vi "config Talon FX.vi"(5 "Reverse Limit switch":T12=enum."Normally Closed", 6 "LIMIT SW\nEnabled?":bool, 7 "Forward Limit switch":T12=enum."Normally Closed", 8 "error in (no error)":errorcluster, 11 "Talon FX motor defaults":T6={"refnum name"="ref DRIVE", "CAN ID"=0, "Installed?"=FALSE, "description"="", "MOTOR SELECT"=0, "CAN Bus"="", "Invert Type"=enum."Counter-Clockwise", "Neutral Mode"=enum."EEPROMSetting", "gear ratio"=0.0, "MOTOR PIDF coefficients"={"PIDF"={"P Gain"=0.001, "I Gain"=0.0, "D Gain"=0.0, "F Gain"=0.0012, "I Zone"=0.0, "Min Output"=-1.0, "Max Output"=1.0}, "Smart Motion"={"Max Velocity"=1900.0, "Max Acceleration"=750.0, "Minimum Velocity Output"=0.1, "Allowed Closed Loop Error"=0.02}}, "Throttle"={"Ramp Open (s)"=0.0, "Ramp Closed (s)"=0.0, "Percent Deadband"=0.0}, "Supply Current Limits"={"Enable?"=FALSE, "Current Limit"=0.0, "Threshold Current"=0.0, "Threshold Time"=0.0}} {"gear ratio" format="%_5f"; "MOTOR SELECT" items=["REV NEO"=5676, "REV NEO 550"=11000, "VEX Falcon"=6380, "WC Kraken"=6000]}) -> (0 "error out":errorcluster, 3 "PhoenixMotorControlDevRef":T1={"DeviceStatus"={"status"=FALSE, "code"=0, "source"=""}, "Type"=enum."PWM", "PWM"={"PWM Channel"=enum."Invalid", "DeadBand"={"Name"="", "maxPositivePwm"=0, "minPositivePwm"=0, "centerPwm"=0, "maxNegativePwm"=0, "minNegativePwm"=0, "angularRange"=0}}, "CAN"={"Device Number"=0, "SetOutput VI Ref"=variant(enum8{"Percent VBus", "Current", "Speed", "Position", "Voltage"} enum."Percent VBus"), "GetOutput VI Ref"=variant(refnum<k1> refnum), "Enable VI Ref"=variant(dbl 12.0), "Disable VI Ref"=variant(enum8{"Percent VBus", "Speed", "Position", "Slave", "Unchanged / Invalid", "Voltage Compensation", "Current", "Motion Profile"} enum."Percent VBus"), "Data"=variant}, "Invert"=FALSE, "DIO PWM"={"PWM \"Enable\" Channel"=enum."Invalid", "DIOChannel"=enum."Invalid", "PWM Rate"=0.0}})   [LabVIEW 2023]
uses:
  ctrl defs/ctrl MOTOR SELECT.ctl
  ctrl defs/ctrl motor PIDF coefficients.ctl
  <vilib>/Rock Robotics/WPI/ThirdParty/REV Robotics/REVLib/Typedef/Spark MAX Smart Motion Parameters.ctl
  <vilib>/Rock Robotics/WPI/ThirdParty/REV Robotics/REVLib/Typedef/Spark MAX Limit Switch Polarity.ctl
  <vilib>/Rock Robotics/WPI/ThirdParty/Phoenix-LabVIEW/Motor Controller/Controls/CTRE_Phoenix_MotorControl_FeedbackDevice_TalonFX.ctl
  <vilib>/Rock Robotics/WPI/ThirdParty/Phoenix-LabVIEW/Motor Controller/Controls/CTRE_Phoenix_MotorControl_TalonFXInvertType.ctl
  <vilib>/Rock Robotics/WPI/ThirdParty/Phoenix-LabVIEW/Motor Controller/Controls/CTRE_Phoenix_MotorControl_NeutralMode.ctl
  ctrl defs/ctrl Talon FX config.ctl
  <vilib>/Rock Robotics/SystemInterfaces/DIO/FPGA_DIOPWMChannel.ctl
  <vilib>/Rock Robotics/WPI/PWM/WPI_PWMDeadband.ctl
  <vilib>/Rock Robotics/WPI/MotorControl/WPI_MotorControlType.ctl
  <vilib>/Rock Robotics/SystemInterfaces/DIO/FPGA_DIOChannel.ctl
  <vilib>/Rock Robotics/WPI/MotorControl/WPI_MotorControlDeviceRef.ctl
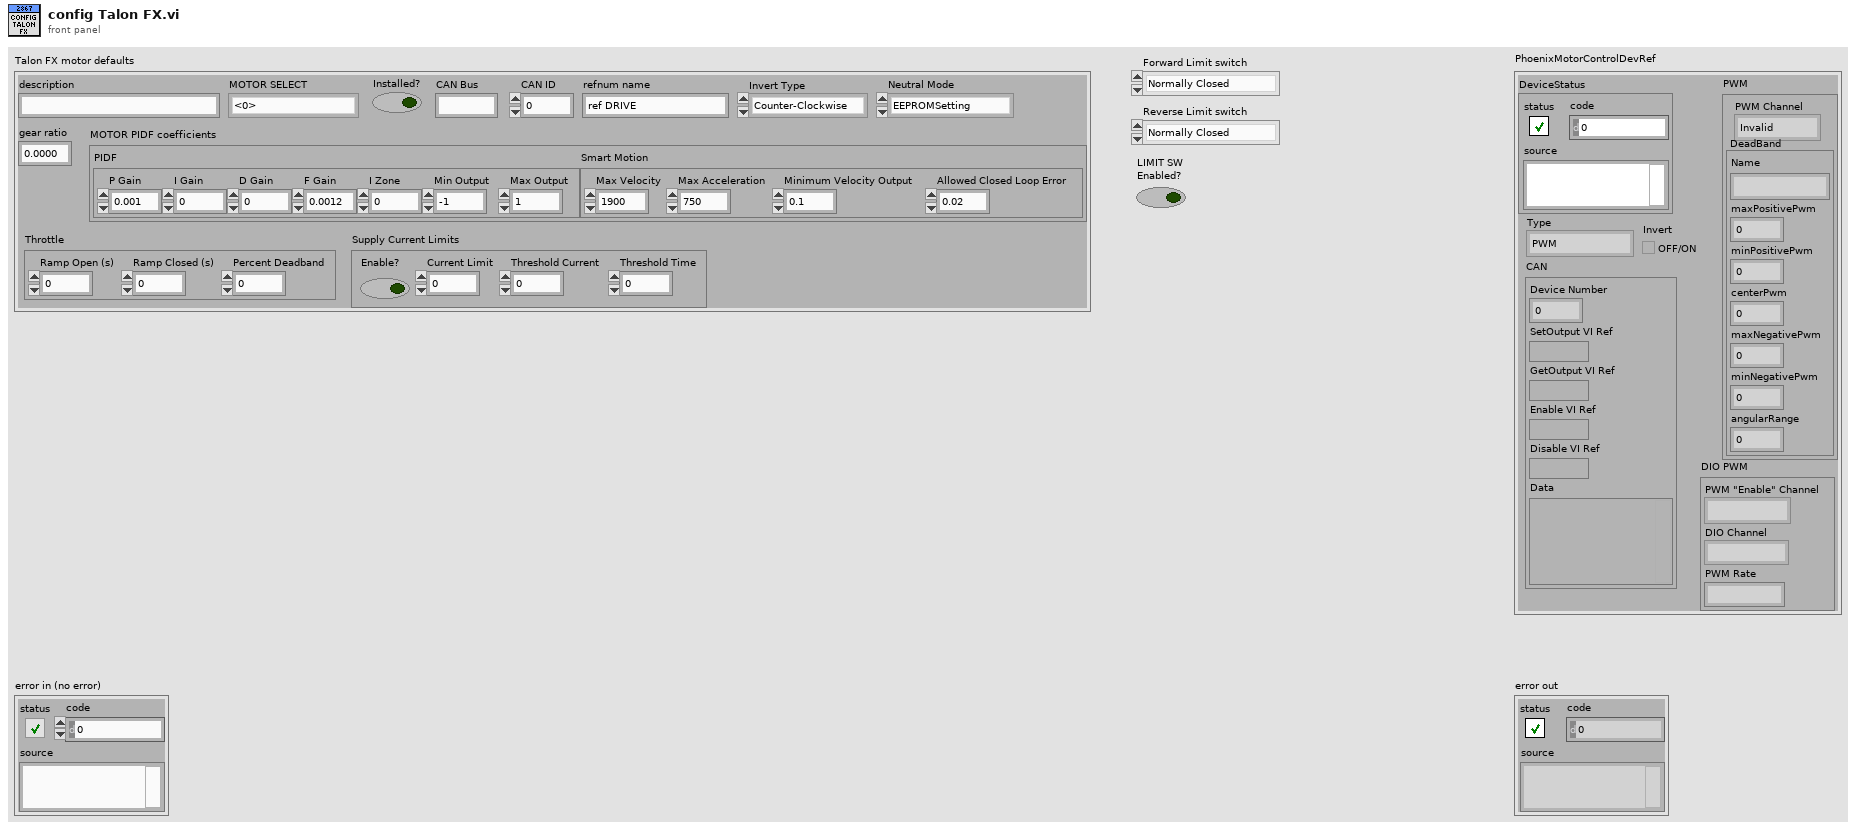
[diagram p1: front panel]
types:
  T1 = typedef "WPI_MotorControlDeviceRef.ctl" = cluster{"DeviceStatus":errorcluster, "Type":T2, "PWM":cluster{"PWM Channel":T3, "DeadBand":T4}, "CAN":cluster{"Device Number":u8, "SetOutput VI Ref":variant, "GetOutput VI Ref":variant, "Enable VI Ref":variant, "Disable VI Ref":variant, "Data":variant}, "Invert":bool, "DIO PWM":cluster{"PWM \"Enable\" Channel":T3, "DIOChannel":T5, "PWM Rate":dbl}}
  T2 = typedef "WPI_MotorControlType.ctl" = enum16{"PWM", "CAN", "DIO PWM"}
  T3 = typedef "FPGA_DIOPWMChannel.ctl" = enum8{"PWM 0", "PWM 1", "PWM 2", "PWM 3", "PWM 4", "PWM 5", "PWM 6", "PWM 7", "PWM 8", "PWM 9", "PWM MXP 0", "PWM MXP 1", "PWM MXP 2", "PWM MXP 3", "PWM MXP 4", "PWM MXP 5", "PWM MXP 6", "PWM MXP 7", "PWM MXP 8", "PWM MXP 9", "Invalid"}
  T4 = typedef "WPI_PWMDeadband.ctl" = cluster{"Name":string, "maxPositivePwm":i32, "minPositivePwm":i32, "centerPwm":i32, "maxNegativePwm":i32, "minNegativePwm":i32, "angularRange":u16}
  T5 = typedef "FPGA_DIOChannel.ctl" = enum8{"DIO 0", "DIO 1", "DIO 2", "DIO 3", "DIO 4", "DIO 5", "DIO 6", "DIO 7", "DIO 8", "DIO 9", "DIO MXP 0", "DIO MXP 1", "DIO MXP 2", "DIO MXP 3", "DIO MXP 4", "DIO MXP 5", "DIO MXP 6", "DIO MXP 7", "DIO MXP 8", "DIO MXP 9", "DIO MXP 10", "DIO MXP 11", "DIO MXP 12", "DIO MXP 13", "DIO MXP 14", "DIO MXP 15", "SPI Port CS1", "SPI Port CS2", "SPI Port CS3", "SPI Port MISO", "SPI Port MOSI", "Invalid"}
  T6 = typedef "ctrl Talon FX config.ctl" = cluster{"refnum name":string, "CAN ID":u8, "Installed?":bool, "description":string, "MOTOR SELECT":T7, "CAN Bus":string, "Invert Type":T8, "Neutral Mode":T9, "gear ratio":dbl, "MOTOR PIDF coefficients":T10, "Throttle":cluster{"Ramp Open (s)":dbl, "Ramp Closed (s)":dbl, "Percent Deadband":dbl}, "Supply Current Limits":cluster{"Enable?":bool, "Current Limit":dbl, "Threshold Current":dbl, "Threshold Time":dbl}}
  T7 = typedef "ctrl MOTOR SELECT.ctl" = i16
  T8 = typedef "CTRE_Phoenix_MotorControl_TalonFXInvertType.ctl" = enum16{"Counter-Clockwise", "Clockwise"}
  T9 = typedef "CTRE_Phoenix_MotorControl_NeutralMode.ctl" = enum8{"EEPROMSetting", "Override to Coast", "Override to Brake"}
  T10 = typedef "ctrl motor PIDF coefficients.ctl" = cluster{"PIDF":cluster{"P Gain":dbl, "I Gain":dbl, "D Gain":dbl, "F Gain":dbl, "I Zone":dbl, "Min Output":dbl, "Max Output":dbl}, "Smart Motion":T11}
  T11 = typedef "Spark MAX Smart Motion Parameters.ctl" = cluster{"Max Velocity":dbl, "Max Acceleration":dbl, "Minimum Velocity Output":dbl, "Allowed Closed Loop Error":dbl}
  T12 = typedef "Spark MAX Limit Switch Polarity.ctl" = enum16{"Normally Open", "Normally Closed"}
  T13 = typedef "CTRE_Phoenix_MotorControl_FeedbackDevice_TalonFX.ctl" = i8
  T14 = cluster{"P Gain":dbl, "I Gain":dbl, "D Gain":dbl, "F Gain":dbl, "I Zone":dbl, "Min Output":dbl, "Max Output":dbl}
  T15 = cluster{"Enable?":bool, "Current Limit":dbl, "Threshold Current":dbl, "Threshold Time":dbl}
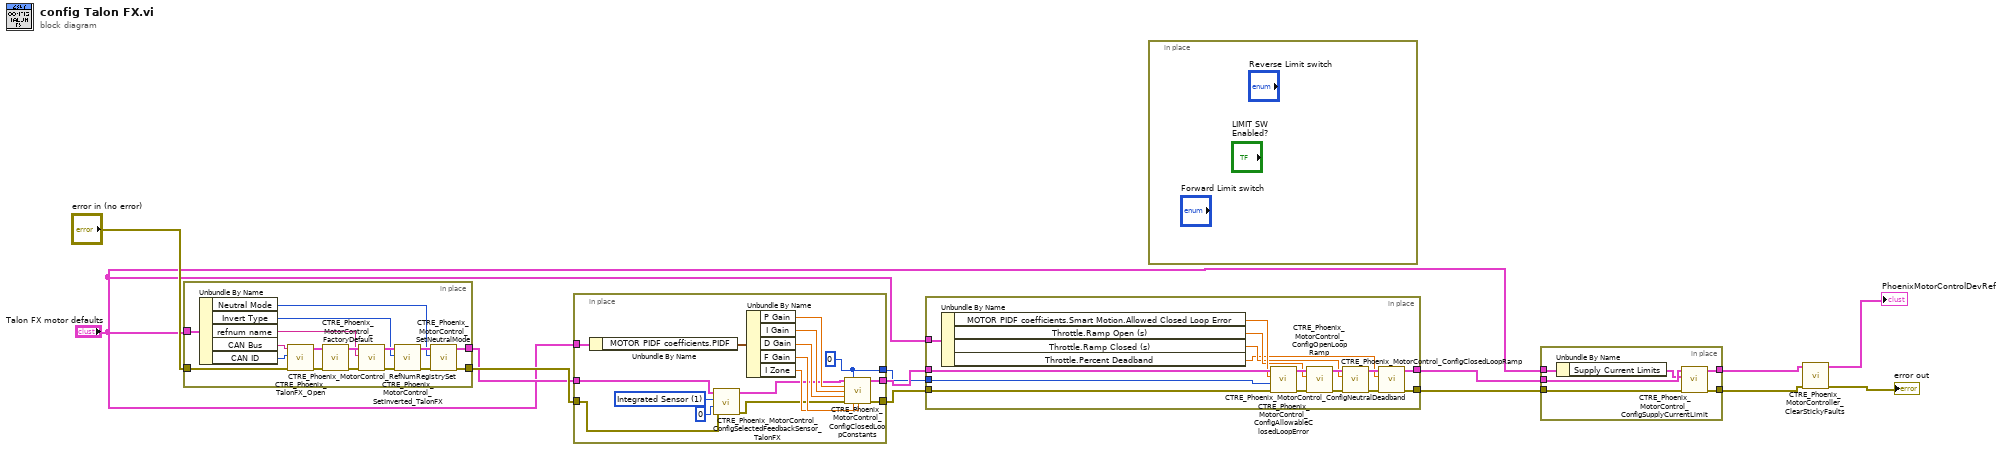
[diagram p0: block diagram]
diagram:
  n1 = in-place {
    in-place-border: "error in (no error)" -> [w22]
    in-place-border: "Talon FX motor defaults" -> [w20]
    in-place-border: [w15] -> w12
    in-place-border: [w14] -> w11
    n2 = Unbundle By Name(w20) -> ("Neutral Mode"=w16:T9, "Invert Type"=w17:T8, "refnum name"=w21:string, "CAN Bus"=w19:string, "CAN ID"=w18:u8)
    n3 = call <vilib>:"CTRE_Phoenix_TalonFX_Open.vi"("error in"=w22, "Device Number"=w18, "CAN Bus"=w19) -> ("error out"=w30:errorcluster, "PhoenixMotorControlDevRef"=w29:T1)  [unwired: 7 in]
    n4 = call <vilib>:"CTRE_Phoenix_MotorControl_FactoryDefault.vi"("error in"=w30, "PhoenixMotorControlDevRef"=w29) -> ("error out"=w25:errorcluster, "PhoenixMotorControlDevRef"=w26:T1)  [unwired: 8 in]
    n5 = call <vilib>:"CTRE_Phoenix_MotorControl_RefNumRegistrySet.vi"("error in (no error)"=w25, "refnum name"=w21, "PhoenixMotorControlDevRef"=w26) -> ("error out"=w23:errorcluster, "PhoenixMotorControlDevRef"=w24:T1)  [unwired: 7 in]
    n6 = call <vilib>:"CTRE_Phoenix_MotorControl_SetInverted_TalonFX.vi"("error in (no error)"=w23, "Invert Type"=w17, "PhoenixMotorControlDevRef"=w24) -> ("error out"=w28:errorcluster, "PhoenixMotorControlDevRef"=w27:T1)  [unwired: 7 in]
    n7 = call <vilib>:"CTRE_Phoenix_MotorControl_SetNeutralMode.vi"("error in (no error)"=w28, "Motor Control Neutral Mode"=w16, "PhoenixMotorControlDevRef"=w27) -> ("error out"=w15:errorcluster, "PhoenixMotorControlDevRef"=w14:T1)  [unwired: 7 in]
  }
  n8 = in-place {
    in-place-border: w12 -> [w33]
    in-place-border: w11 -> [w34]
    in-place-border: [w46] -> w10
    in-place-border: [w45] -> w9
    in-place-border: "Talon FX motor defaults" -> [w44]
    in-place-border: [w37] -> w8
    w35 = T13 1 items=["Integrated Sensor"=1, "Sensor Sum (S0 + S1)"=9, "Sensor Difference (D0 - D1)"=10, "Remote Source 0"=11, "Remote Source 1"=12, "None"=14, "Software Emulated"=15] ("Talon FX Feedback Device")
    w37 = 0 ("slotIdx")
    n9 = Unbundle By Name(w44) -> ("MOTOR PIDF coefficients.PIDF"=w43:T14)
    n10 = call <vilib>:"CTRE_Phoenix_MotorControl_ConfigSelectedFeedbackSensor_TalonFX.vi"("error in (no error)"=w33, "pidLoopIdx"=0, "Talon FX Feedback Device"=w35, "PhoenixMotorControlDevRef"=w34) -> ("error out"=w31:errorcluster, "PhoenixMotorControlDevRef"=w32:T1)  [unwired: 6 in]
    n11 = Unbundle By Name(w43) -> ("P Gain"=w42:dbl, "I Gain"=w41:dbl, "D Gain"=w40:dbl, "F Gain"=w39:dbl, "I Zone"=w38:dbl)
    n12 = call <vilib>:"CTRE_Phoenix_MotorControl_ConfigClosedLoopConstants.vi"("PhoenixMotorControlDevRef"=w32, "slotIdx"=w37, "P"=w42, "I"=w41, "D"=w40, "error in (no error)"=w31, "F"=w39, "I Zone"=w38) -> ("PhoenixMotorControlDevRef"=w45:T1, "error out"=w46:errorcluster)  [unwired: 6 in]
  }
  n13 = in-place {
    in-place-border: w10 -> [w56]
    in-place-border: w9 -> [w55]
    in-place-border: "Talon FX motor defaults" -> [w53]
    in-place-border: w8 -> [w54]
    in-place-border: [w48] -> w6
    in-place-border: [w47] -> w7
    n14 = Unbundle By Name(w53) -> ("MOTOR PIDF coefficients.Smart Motion.Allowed Closed Loop Error"=w52:dbl, "Throttle.Ramp Open (s)"=w51:dbl, "Throttle.Ramp Closed (s)"=w50:dbl, "Throttle.Percent Deadband"=w49:dbl)
    n15 = call <vilib>:"CTRE_Phoenix_MotorControl_ConfigAllowableClosedLoopError.vi"("error in (no error)"=w56, "slotIdx"=w54, "allowableClosedLoopError"=w52, "PhoenixMotorControlDevRef"=w55) -> ("error out"=w62:errorcluster, "PhoenixMotorControlDevRef"=w61:T1)  [unwired: 6 in]
    n16 = call <vilib>:"CTRE_Phoenix_MotorControl_ConfigOpenLoopRamp.vi"("error in (no error)"=w62, "secondsFromNeutralToFull"=w51, "PhoenixMotorControlDevRef"=w61) -> ("error out"=w60:errorcluster, "PhoenixMotorControlDevRef"=w59:T1)  [unwired: 7 in]
    n17 = call <vilib>:"CTRE_Phoenix_MotorControl_ConfigClosedLoopRamp.vi"("error in (no error)"=w60, "secondsFromNeutralToFull"=w50, "PhoenixMotorControlDevRef"=w59) -> ("error out"=w58:errorcluster, "PhoenixMotorControlDevRef"=w57:T1)  [unwired: 7 in]
    n18 = call <vilib>:"CTRE_Phoenix_MotorControl_ConfigNeutralDeadband.vi"("error in (no error)"=w58, "Percent Deadband"=w49, "PhoenixMotorControlDevRef"=w57) -> ("error out"=w48:errorcluster, "PhoenixMotorControlDevRef"=w47:T1)  [unwired: 7 in]
  }
  n19 = in-place {
  }
  n20 = in-place {
    in-place-border: w7 -> [w68]
    in-place-border: w6 -> [w67]
    in-place-border: "Talon FX motor defaults" -> [w66]
    in-place-border: [w64] -> w4
    in-place-border: [w63] -> w3
    n21 = Unbundle By Name(w66) -> ("Supply Current Limits"=w65:T15)
    n22 = call <vilib>:"CTRE_Phoenix_MotorControl_ConfigSupplyCurrentLimit.vi"("error in (no error)"=w67, "Supply Current Limit Configuration"=w65, "PhoenixMotorControlDevRef"=w68) -> ("error out"=w63:errorcluster, "PhoenixMotorControlDevRef"=w64:T1)  [unwired: 7 in]
  }
  n23 = call <vilib>:"CTRE_Phoenix_MotorController_ClearStickyFaults.vi"("error in"=w3, "PhoenixMotorControlDevRef"=w4) -> ("error out"=→"error out":errorcluster, "PhoenixMotorControlDevRef"=→"PhoenixMotorControlDevRef":T1)  [unwired: 8 in]
